vi "HEWH Thermal Eff Coerce.vi"(8 "error in (no error)":errorcluster, 11 "Eff Input":dbl min=0.0 max=1.0) -> (0 "error out":errorcluster, 3 "Eff Output":dbl)   [LabVIEW 2016]
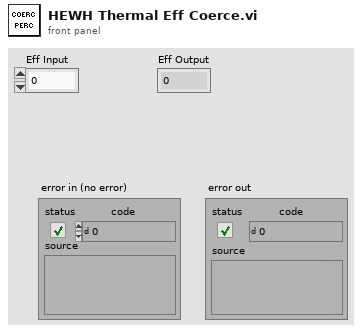
[diagram p1: front panel]
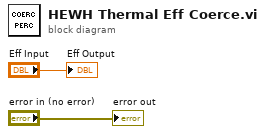
[diagram p0: block diagram]
diagram:
  "Eff Output" <- "Eff Input"
  "error out" <- "error in (no error)"
